vi "Close_Data_Trans_Ref.vi"() -> (0 "Error Out":errorcluster)   [LabVIEW 2011]
uses:
  DataTranslation_global.vi
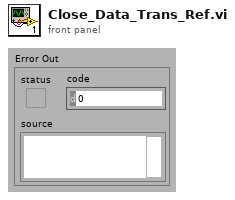
[diagram p1: front panel]
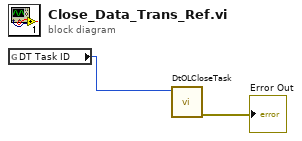
[diagram p0: block diagram]
diagram:
  n1 = global read "DataTranslation_global.vi" "DT Task ID"() -> (w1:i32)
  n2 = call <userlib>:"DtOLCloseTask.vi"("Task in"=w1) -> ("Error Out"=→"Error Out":errorcluster)  [unwired: 10 in]
